vi "Aux TE Controllers Serial Write and Read.vi"(4 "second string":string, 6 "error in":errorcluster, 7 "Action":T2, 8 "string to write":string, 9 "TE Controller Serial Ports In":T1[](array[typedef]) {"XOFF Char" format="%.0x"; "XON Char" format="%.0x"; "flow control" items=["None"=0, "XON/XOFF"=1, "RTS/CTS"=2, "DTR/DSR"=4]; "stop bits" items=["1.0"=10, "1.5"=15, "2.0"=20]; "baud rate" items=["1.0"=10, "1.5"=15, "2.0"=20]; "termination char" format="%.0x"}) -> (0 "Error Out":errorcluster, 1 "#Bytes R/W":i16[](array[numeric]), 2 "Data Read":string[](array[string]), 3 "TE Controller Serial Ports Out":T1[](array[typedef]) {"XOFF Char" format="%.0x"; "XON Char" format="%.0x"; "flow control" items=["None"=0, "XON/XOFF"=1, "RTS/CTS"=2, "DTR/DSR"=4]; "stop bits" items=["1.0"=10, "1.5"=15, "2.0"=20]; "baud rate" items=["1.0"=10, "1.5"=15, "2.0"=20]; "termination char" format="%.0x"}, 5 "appended array":string[](array[string]))   [LabVIEW 2016]
doc: "The Advanced Serial Read and Write example performs a Serial Port Read, a Serial Port Write, or a combination of these actions while setting some advanced serial features like buffer size, termination characters, and XON/XOFF flow control. The user selects the actions (read or write) on the front panel. If both are selected, the VI will write the data first, read the data and then close the VISA session that is opened to the port. \n\nThe parameters set for the serial port must match the parameters of the connected instrument or device. In this example, the bytes to read parameter specifies the number of bytes that the serial port reads. If there were more bytes at the port than the number specified in bytes to read, those bytes would not be read. Also, if you specify to read more bytes than the number of bytes actually read, you might receive a timeout error message.\n\nINSTRUCTIONS:\n1) Select the serial resource and configuration parameters (baud rate, data bits, parity, stop bits, flow control).\n2) Termination character can be enabled and set. Also, set the required input buffer size prior to running the example.\n3) Select the operations to be performed. \n4) Connect the serial port to your device. If no device is available, perform a loopback test by doing one of the following. Short pins 2 and 3 on a RS-232 cable or short pin 4 to pin 8 and pin 5 to pin 9 on a RS-485/422 cable. \n5) Run the VI to see the data read. (The \"read string\" will match the \"string to write\" if a loopback test was performed.)\n\nThis example exposes several advanced features that you may need for your application. Not all applications need all the features shown in this example. The input buffer size is likely an important setting that you want to control in your application. This example expands upon the flow control option for XON and XOFF, allowing the user to choose those control characters. The timeout parameter has been brought to the front panel so a user can specify the time period the VISA Read will wait for the number of bytes to read before timing out. Also, the user has several controls for the termination character, which is discussed later.\n\nNote that you can press the write and read buttons and change the bytes to read parameters on the fly, while the example is running. However, you must stop the example to change the other configuration parameters after the example has started running, and then run again.\n\nSet the I/O buffer size slightly higher the amount of data you expect to receive. This is very important for applications that don't use flow control, as you may lose characters if the receive buffer overflows.\n\nSetting the timeout period ensures that the operation returns with a timeout error if the operation cannot be performed in the specified time period. \n\nSome devices require a termination character in order to identify the end of command strings. Some devices send a termination character to signify the end of data to be read. \n\nThis example shows how you can end the Read operation once a termination character is detected in the buffer and/or append a termination character at the end of the Write data. To enable the Read to end on a termination character, use the VISA Configure Serial Port or use the VISA Properties Serial End Mode for Reads, Termination Character Enable, and Termination Character. To end the Write with a termination character, use the VISA Properties Serial End Mode for Writes, the Send End Enable, and Termination Character. In this example, the same termination character is used for both the Read and the Write. You can specify two different characters for your application, if desired.\n\nYour application may require specific characters for the XON/XOFF Flow Control. You can specify these characters with the VISA Properties Flow Control XOFF Character and Flow Control XON Character. Note that if the standard XON and XOFF characters are used, then decimal 17 and 19 are unavailable for data values. Remember that using flow control and setting an adequate buffer size allow you to prevent buffer overflows."
uses:
  Controls/SerialPortControl.ctl
  Controls/Serial Visa Control.ctl
  <vilib>/Instr/_visa.llb/VISA Configure Serial Port (Instr).vi
panel:
  # "Select the serial resource and the operations to be performed.  If all are selected, the VI will write the data first, read data and then close the VISA session that is opened to the port.  This VI will wait until the specified number of bytes is received at the port until the timeout period is met.  Only the specified number of bytes will be read unless the read ends on a termination character.  The termination character can be enabled and set.  Also, set the required input buffer size prior to running the example.\nNote: The example loops until the STOP button is pressed."
  # "For additional information select File >> VI Properties >> Documentation"
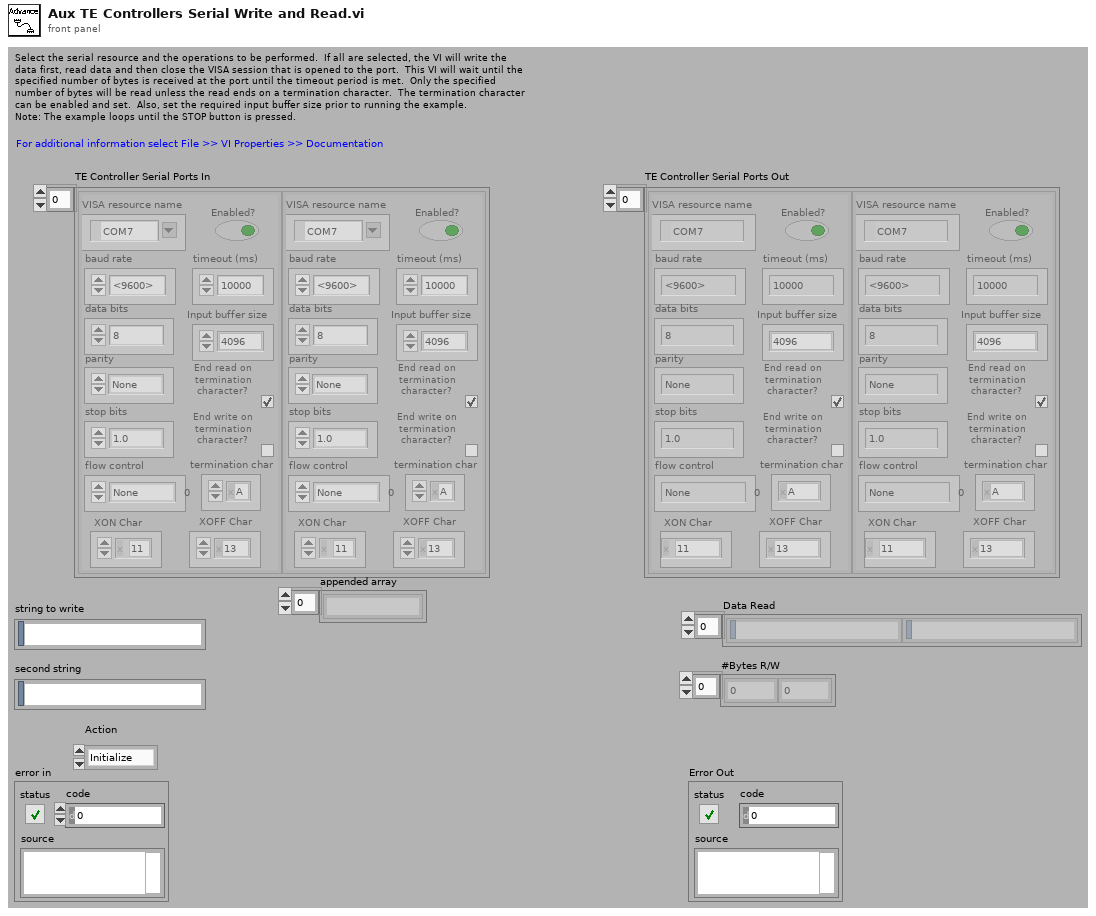
[diagram p1: front panel]
types:
  T1 = typedef "Serial Visa Control.ctl" = cluster{"termination char":u8, "End read on termination character?":bool, "Enabled?":bool, "VISA resource name":refnum<visa-resource-name>, "baud rate":u32, "data bits":u16, "parity":enum16{"None", "Odd", "Even", "Mark", "Space"}, "stop bits":u16, "flow control":u16, "timeout (ms)":u32, "Input buffer size":u32, "End write on termination character?":bool, "XON Char":u8, "XOFF Char":u8}
  T2 = typedef "SerialPortControl.ctl" = enum16{"Initialize", "Write Data", "Read Data", "Close Port"}
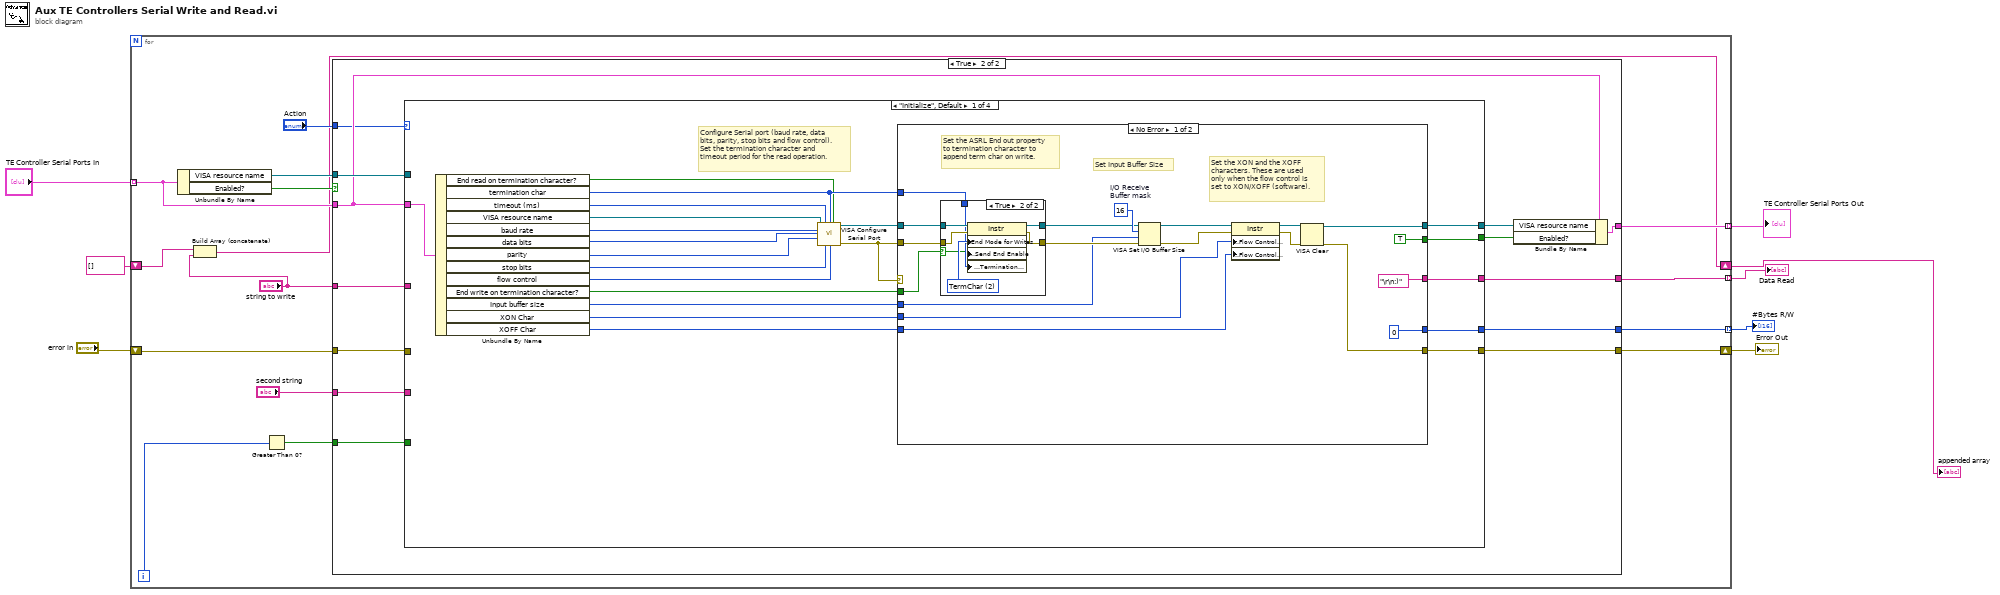
[diagram p0: block diagram]
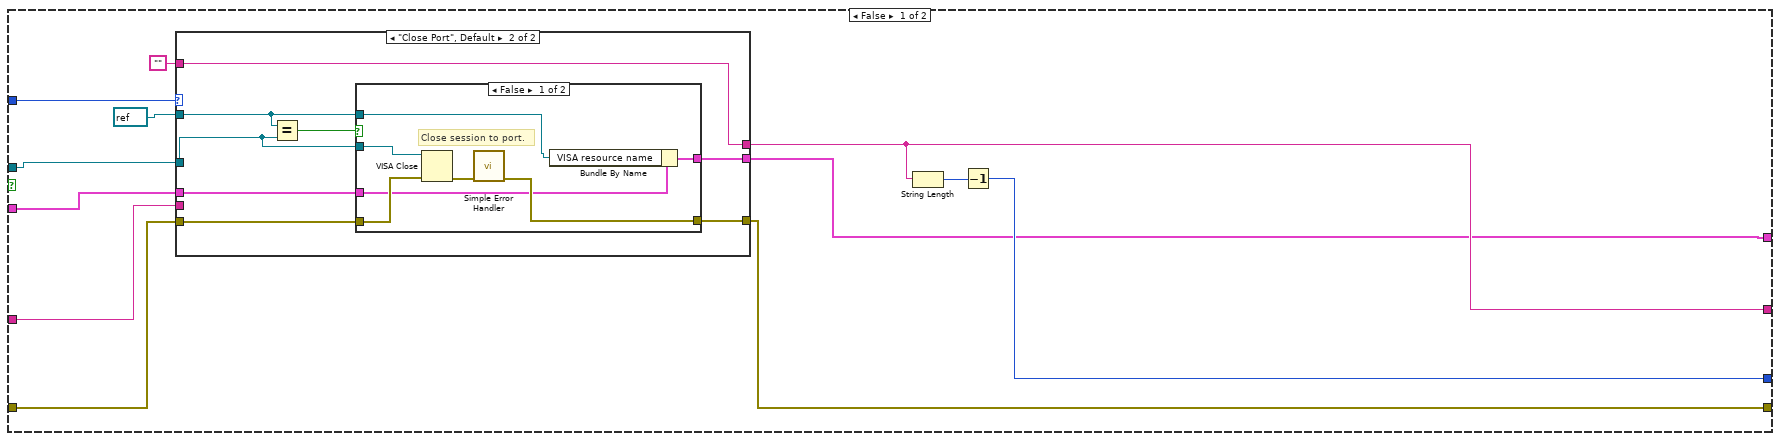
[diagram p2: hidden frame]
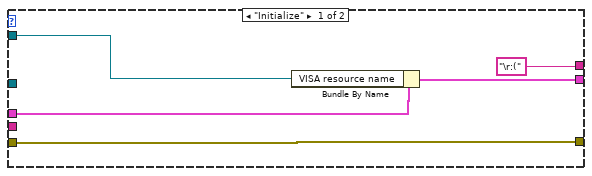
[diagram p3: hidden frame]
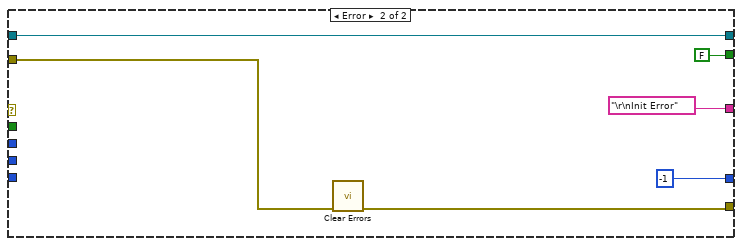
[diagram p6: hidden frame]
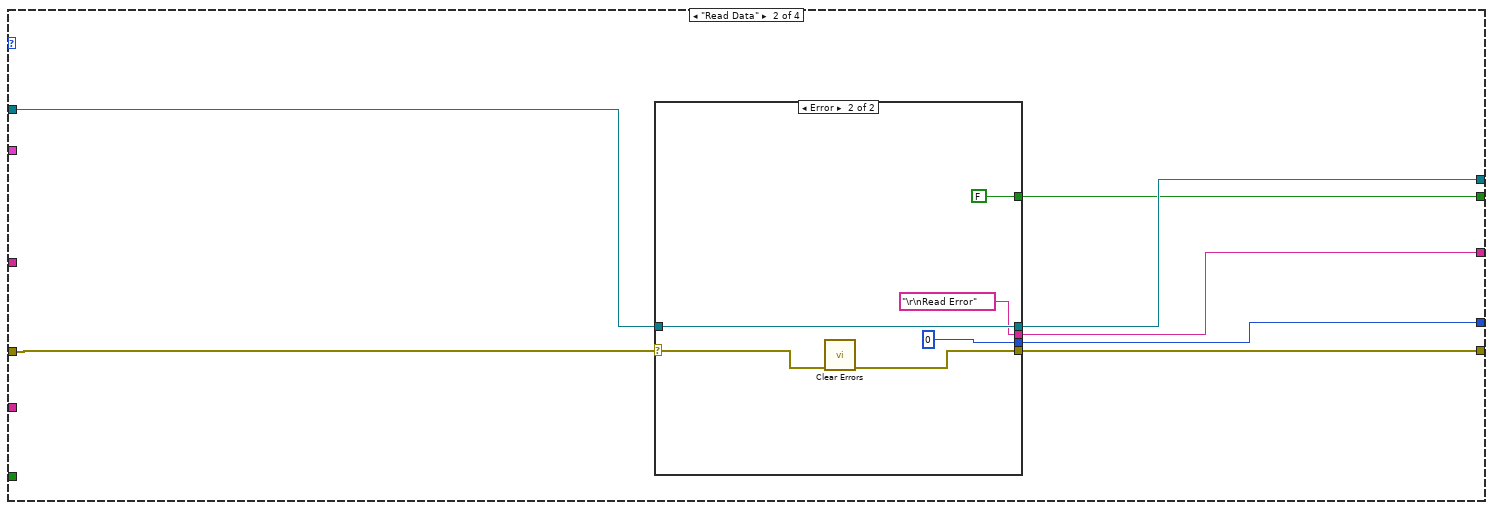
[diagram p7: hidden frame]
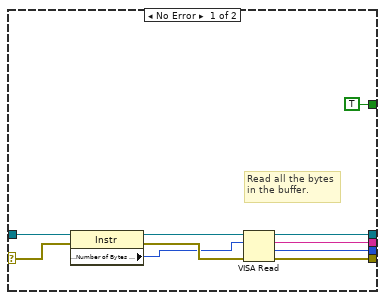
[diagram p8: hidden frame]
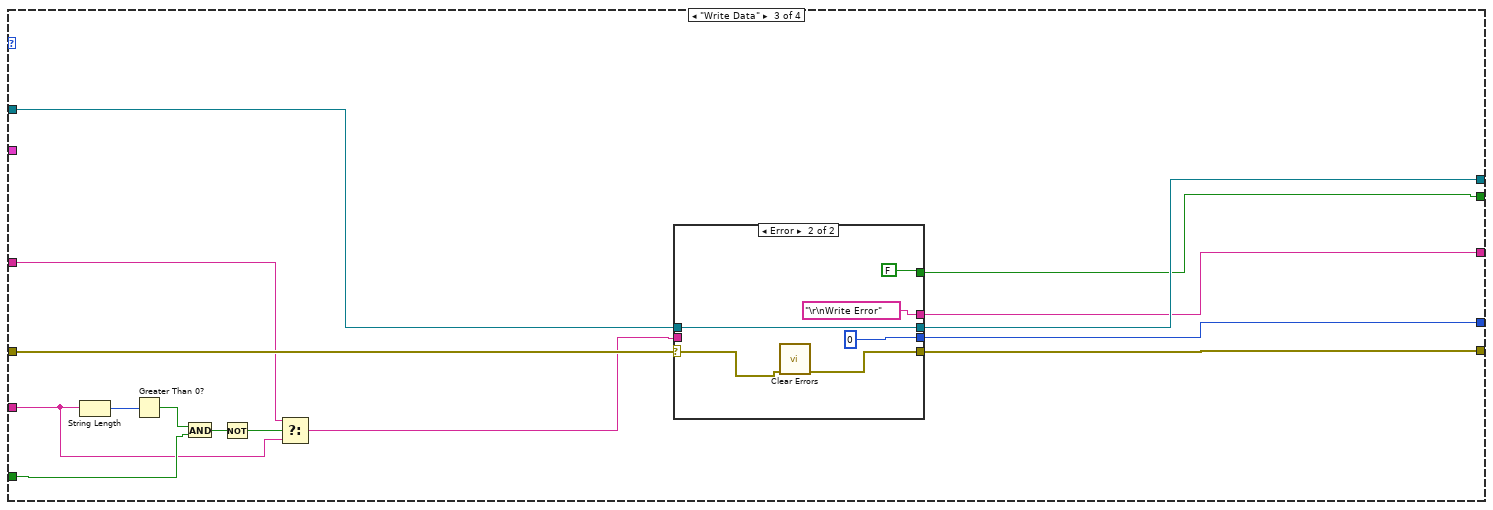
[diagram p9: hidden frame]
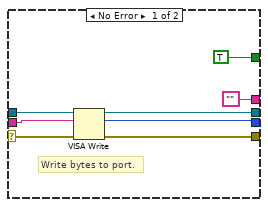
[diagram p10: hidden frame]
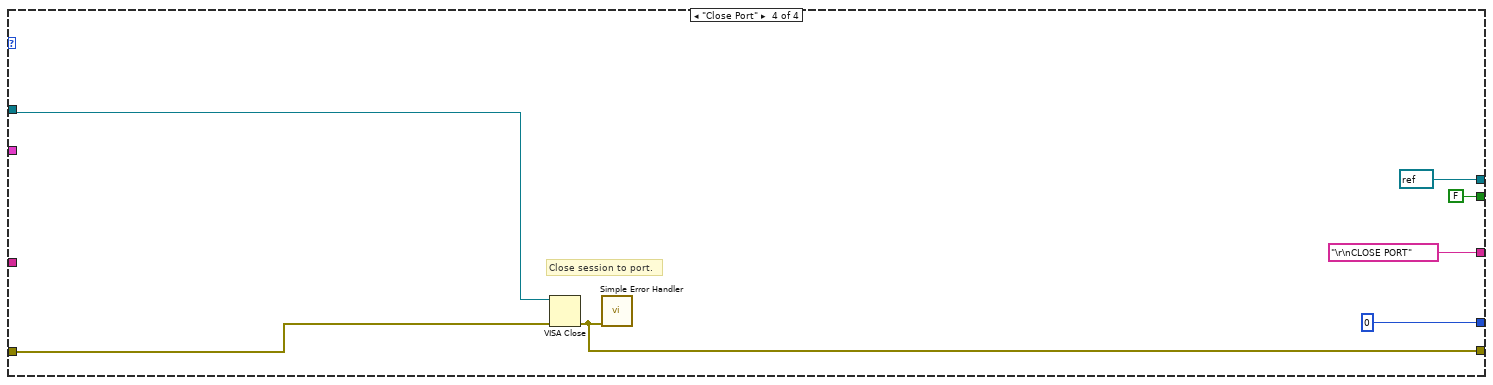
[diagram p11: hidden frame]
diagram:
  n1 = for {
    tunnel: "TE Controller Serial Ports In" -> [w21] mode=indexing
    shift-right: [w18] -> w6
    shift-left: "error in" -> [w20]
    tunnel: [w19] -> w5 mode=indexing
    tunnel: [w17] -> w4 mode=indexing
    tunnel: [w16] -> w3 mode=indexing
    shift-right: [w9] -> w1
    shift-left: string[] [] -> [w10]
    i -> [w14]
    n2 = Unbundle By Name(w21) -> ("VISA resource name"=w23:refnum<visa-resource-name>, "Enabled?"=w22:bool)
    n3 = Build Array (concatenate)(w10, "string to write") -> (w9:string[])
    n4 = Greater Than 0?(x=w14) -> (x > 0?=w13:bool)
    n5 = case shown="True" w22 {
      tunnel: w20 -> [w27 w70]
      tunnel: w23 -> [w29 w69]
      tunnel: w21 -> [w28 w65]
      tunnel: [w25 w67] -> w19
      tunnel: [w26 w66] -> w18
      tunnel: [w30 w63] -> w17
      tunnel: [w32 w62] -> w16
      tunnel: "Action" -> [w35 w61]
      tunnel: "string to write" -> [w33 w60]
      tunnel: w13 -> [_ w59]
      tunnel: "second string" -> [_ w58]
      frame False {
        n6 = case shown="\"Close Port\", Default" w35 {
          tunnel: "" -> [_ w48]
          tunnel: ["\r:(" w48] -> w32
          tunnel: w33 -> [_ _]
          tunnel: w29 -> [_ w44]
          tunnel: w28 -> [w38 w46]
          tunnel: [w37 w45] -> w25
          tunnel: w27 -> [w39 w43]
          tunnel: [w39 w42] -> w26
          tunnel: refnum<visa-resource-name> refnum ("VISA resource name") -> [w36 w41]
          frame "Initialize" {
            n7 = Bundle By Name(cluster=w38, "VISA resource name"=w36) -> (w37:T1)
          }
          frame "Close Port", Default {
            n8 = Equal?(x=w41, y=w44) -> (x = y?=w47:bool)
            n9 = case shown="False" w47 {
              tunnel: [w51 w57] -> w45
              tunnel: w46 -> [w50 w57]
              tunnel: w41 -> [w49 _]
              tunnel: w44 -> [w54 _]
              tunnel: w43 -> [w53 w56]
              tunnel: [w52 w56] -> w42
              frame False {
                # "Close session to port."
                n10 = VISA Close(VISA resource name=w54, error in (no error)=w53) -> (error out=w55:errorcluster)
                n11 = call <vilib>:"Simple Error Handler.vi"("error in (no error)"=w55) -> ("error out"=w52:errorcluster)  [unwired: 4 in, 4 out]
                n12 = Bundle By Name(cluster=w50, "VISA resource name"=w49) -> (w51:T1)
              }
              frame True {
              }
            }
          }
        }
        n13 = String Length(string=w32) -> (length=w31:i32)
        n14 = Decrement(x=w31) -> (x-1=w30:i32)
      }
      frame True {
        n15 = case shown="\"Initialize\", Default" w61 {
          tunnel: [w91 w131 w163 w182] -> w66
          tunnel: [w89 w132 w162 refnum<visa-resource-name> refnum ("VISA resource name")] -> w68
          tunnel: w69 -> [_ w130 w161 w184]
          tunnel: w70 -> [_ w129 w160 w183]
          tunnel: w65 -> [w75 _ _ _]
          tunnel: [w73 w128 w159 FALSE] -> w64
          tunnel: [w72 w126 w158 u32 0 ("return count")] -> w63
          tunnel: [w71 w127 w157 "\r\nCLOSE PORT"] -> w62
          tunnel: w60 -> [_ _ w150 _]
          tunnel: w59 -> [_ _ w154 _]
          tunnel: w58 -> [_ _ w151 _]
          frame "Initialize", Default {
            # "Configure Serial port (baud rate, data\nbits, parity, stop bits and flow control).\nSet the termination character and\ntimeout period for the read operation."
            n16 = Unbundle By Name(w75) -> ("End read on termination character?"=w80:bool, "termination char"=w81:u8, "timeout (ms)"=w82:u32, "VISA resource name"=w88:refnum<visa-resource-name>, "baud rate"=w87:u32, "data bits"=w86:u16, "parity"=w85:enum16{"None", "Odd", "Even", "Mark", "Space"}, "stop bits"=w84:u16, "flow control"=w83:u16, "End write on termination character?"=w79:bool, "Input buffer size"=w78:u32, "XON Char"=w77:u8, "XOFF Char"=w76:u8)
            n17 = call-poly "VISA Configure Serial Port"("VISA resource name"=w88, "timeout (10sec)"=w82, "termination char\n(0xA = '\\n' = LF)"=w81, "Enable Termination\nChar (T)"=w80, "baud rate (9600)"=w87, "data bits (8)"=w86, "parity (0:none)"=w85, "stop bits (10: 1 bit)"=w84, "flow control (0:none)"=w83) -> ("VISA resource name out"=w90:refnum<visa-resource-name>, "error out"=w74:errorcluster)  [unwired: 5 in]
            n18 = case shown="No Error" w74 {
              tunnel: [w92 w123] -> w91
              tunnel: w74 -> [w107 w122]
              tunnel: w90 -> [w104 w124]
              tunnel: [w94 w124] -> w89
              tunnel: w81 -> [w103 _]
              tunnel: w79 -> [w102 _]
              tunnel: w78 -> [w101 _]
              tunnel: w77 -> [w100 _]
              tunnel: w76 -> [w99 _]
              tunnel: [TRUE FALSE] -> w73
              tunnel: [0 -1] -> w72
              tunnel: ["\r\n:)" "\r\nInit Error"] -> w71
              frame No Error {
                w110 = u16 16  # I/O Receive Buffer mask
                # "Set the XON and the XOFF\ncharacters. These are used\nonly when the flow control is\nset to XON/XOFF (software)."
                # "Set Input Buffer Size"
                # "Set the ASRL End out property\nto termination character to\nappend term char on write."
                n19 = case shown="True" w102 {
                  selector: w102 -> [_ w113]
                  tunnel: w104 -> [w111 w119]
                  tunnel: w107 -> [w112 w118]
                  tunnel: [w111 w117] -> w105
                  tunnel: [w112 w116] -> w106
                  tunnel: w103 -> [_ w114]
                  frame False {
                  }
                  frame True {
                    w115 = u16 2 items=["None", "LastBit", "TermChar", "Break"] ("Serial Settings:Serial End Mode for Writes")
                    n20 = property class="Instr"(reference=w119, error in=w118, "Serial Settings:End Mode for Writes"=w115, "Message Based Settings:Send End Enable"=w113, "Message Based Settings:Termination Character"=w114) -> (reference out=w117:refnum<visa-resource-name>, error out=w116:errorcluster)
                  }
                }
                n21 = VISA Set I/O Buffer Size(VISA resource name=w105, mask (16)=w110, size (4096)=w101, error in (no error)=w106) -> (VISA resource name out=w109:refnum<visa-resource-name>, error out=w108:errorcluster)
                n22 = property class="Instr"(reference=w109, error in=w108, "Serial Settings:Flow Control XON Character"=w100, "Serial Settings:Flow Control XOFF Character"=w99) -> (reference out=w95:refnum<visa-resource-name>, error out=w93:errorcluster)
                n23 = VISA Clear(VISA resource name=w95, error in (no error)=w93) -> (VISA resource name out=w94:refnum<visa-resource-name>, error out=w92:errorcluster)
              }
              frame Error {
                n24 = call <vilib>:"Clear Errors.vi"("error in (no error)"=w122) -> ("error out"=w123:errorcluster)  [unwired: 5 in, 1 out]
              }
            }
          }
          frame "Read Data" {
            n25 = case "Read bytes from port." shown="Error" w129 {
              selector: w129 -> [w133 w147]
              tunnel: [w141 w146] -> w131
              tunnel: [w142 w148] -> w132
              tunnel: w130 -> [w137 w148]
              tunnel: [TRUE FALSE] -> w128
              tunnel: [w139 "\r\nRead Error"] -> w127
              tunnel: [w138 u32 0 ("return count")] -> w126
              frame No Error {
                # "Read all the bytes\nin the buffer."
                n26 = property class="Instr"(reference=w137, error in=w133) -> (reference out=w136:refnum<visa-resource-name>, error out=w135:errorcluster, "Serial Settings:Number of Bytes at Serial Port"=w134:u32)
                n27 = VISA Read(VISA resource name=w136, byte count=w134, error in (no error)=w135) -> (VISA resource name out=w142:refnum<visa-resource-name>, read buffer=w139:string, return count=w138:u32, error out=w141:errorcluster)
              }
              frame Error {
                # "Error occurred \nreading Bytes at \nSerial Port"
                n28 = call <vilib>:"Clear Errors.vi"("error in (no error)"=w147) -> ("error out"=w146:errorcluster)  [unwired: 5 in, 1 out]
              }
            }
          }
          frame "Write Data" {
            n29 = String Length(string=w151) -> (length=w156:i32)
            n30 = Greater Than 0?(x=w156) -> (x > 0?=w155:bool)
            n31 = And(x=w155, y=w154) -> (x .and. y?=w153:bool)
            n32 = Not(x=w153) -> (.not. x?=w152:bool)
            n33 = Select(t=w150, s=w152, f=w151) -> (s? t:f=w149:string)
            n34 = case shown="Error" w160 {
              selector: w160 -> [w168 w174]
              tunnel: [w171 w177] -> w162
              tunnel: [w170 w175] -> w163
              tunnel: w161 -> [w169 w177]
              tunnel: [TRUE FALSE] -> w159
              tunnel: [w166 u32 0 ("return count")] -> w158
              tunnel: ["" "\r\nWrite Error"] -> w157
              tunnel: w149 -> [w164 _]
              frame No Error {
                # "Write bytes to port."
                n35 = VISA Write(VISA resource name=w169, write buffer=w164, error in (no error)=w168) -> (VISA resource name out=w171:refnum<visa-resource-name>, return count=w166:u32, error out=w170:errorcluster)
              }
              frame Error {
                n36 = call <vilib>:"Clear Errors.vi"("error in (no error)"=w174) -> ("error out"=w175:errorcluster)  [unwired: 5 in, 1 out]
              }
            }
          }
          frame "Close Port" {
            # "Close session to port."
            n37 = VISA Close(VISA resource name=w184, error in (no error)=w183) -> (error out=w182:errorcluster)
            n38 = call <vilib>:"Simple Error Handler.vi"("error in (no error)"=w182) -> ()  [unwired: 4 in, 5 out]
          }
        }
        n39 = Bundle By Name(cluster=w65, "VISA resource name"=w68, "Enabled?"=w64) -> (w67:T1)
      }
    }
  }
  "Error Out" <- w6
  "TE Controller Serial Ports Out" <- w5
  "#Bytes R/W" <- w4
  "Data Read" <- w3
  "appended array" <- w1
